vi "PH_Acq_ms.vi"(2 "PH_Settings_Params":T1={"SyncDiv"=1, "DeviceIndex"=0, "CFD0 level"=50, "CFD0 zero X"=10, "CFD1 level"=50, "CFD1 zero X"=10, "Range No."=0, "StopOnOverflow"=FALSE, "AcqTime (ms)"=0.0} {"Range No." min=0 max=5 step=1; "CFD1 zero X" min=0 max=40 step=1; "CFD1 level" min=0 max=400 step=1; "CFD0 zero X" min=-1300 max=400 step=10; "CFD0 level" min=-1300 max=400 step=10; "SyncDiv" min=1 max=8 step=1}, 3 "Deviceindex":i32, 4 "Calib Error":bool, 5 "Initialization Error":bool) -> (0 "CH1MeanRate":dbl format="%0.2f", 1 "SyncMeanRate":dbl format="%0.2f")   [LabVIEW 2019]
uses:
  <vilib>/Analysis/baseanly.llb/Mean (DBL).vi
  phlib64.dll
  <vilib>/Analysis/NI_AALBase.lvlib
panel:
  out "Elapsed Time (s)":dbl
  out "CH1Rates":i32[](array[numeric])
  out "SyncRates":i32[](array[numeric])
  out "Waveform Chart":cluster{"rate":i32}[](graph)
  out "CH1Rate":i32(slide) scale=1.0..1000000.0
  out "SyncRate":i32(slide) scale=1.0..1000000.0
  in  "stop":bool
  out "Resolution (ps)":i32
  out "PH_Settings_Error":bool
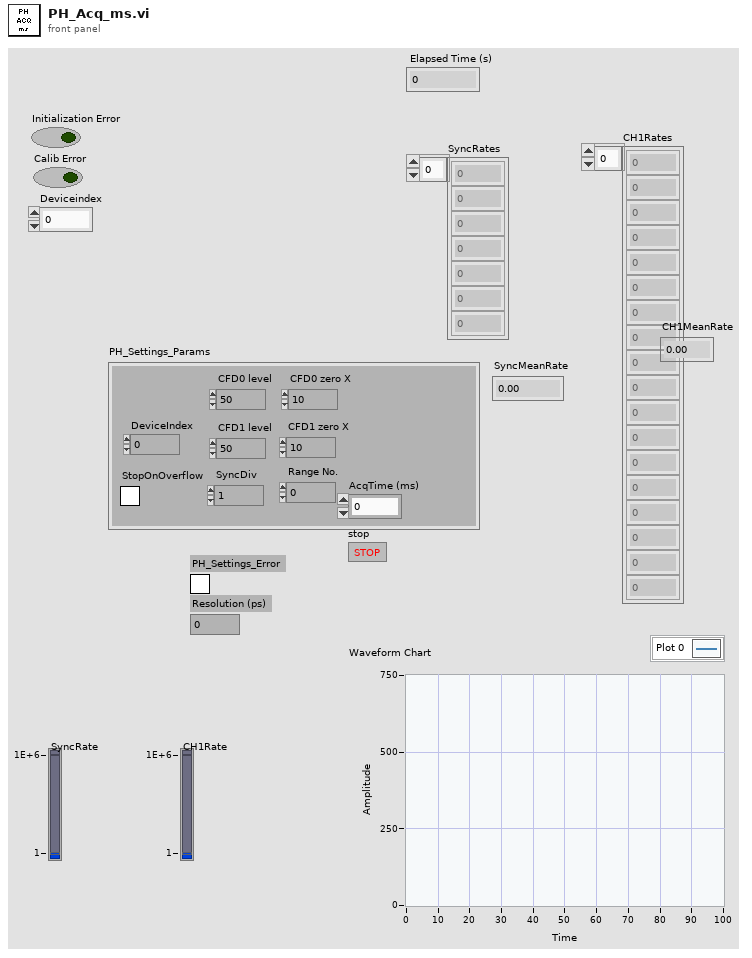
[diagram p1: front panel]
types:
  T1 = cluster{"SyncDiv":i32, "DeviceIndex":i32, "CFD0 level":i32, "CFD0 zero X":i32, "CFD1 level":i32, "CFD1 zero X":i32, "Range No.":i32, "StopOnOverflow":bool, "AcqTime (ms)":dbl}
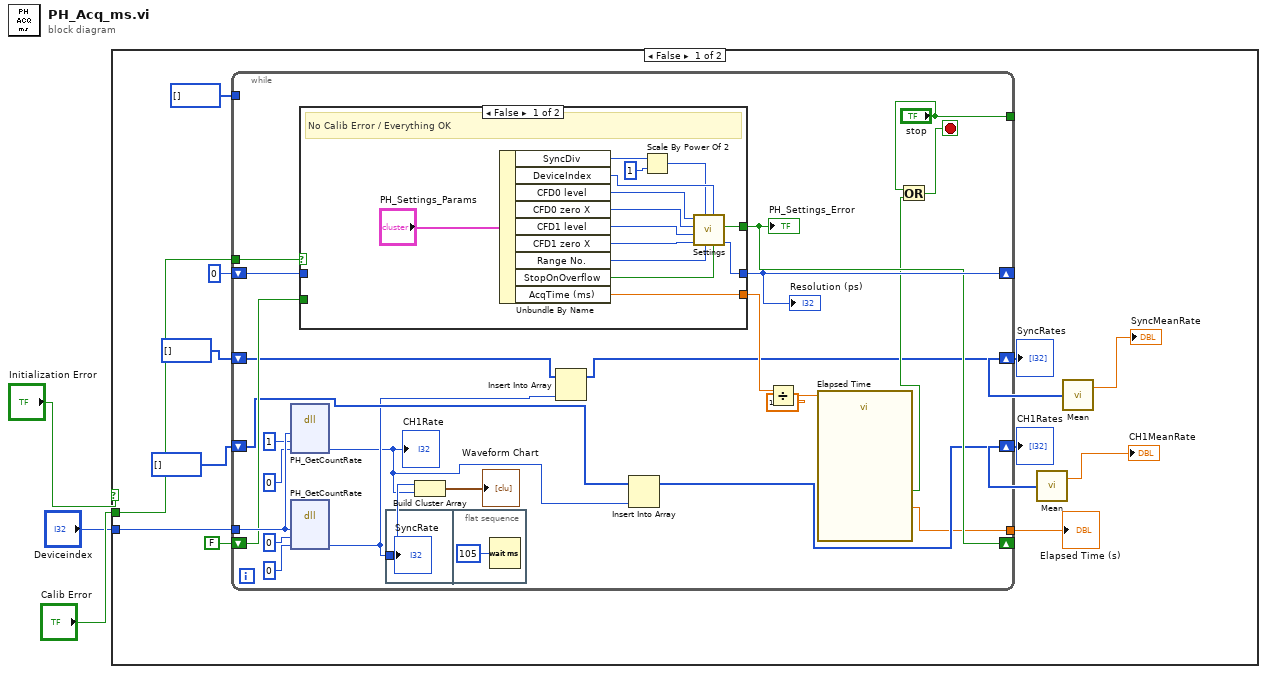
[diagram p0: block diagram]
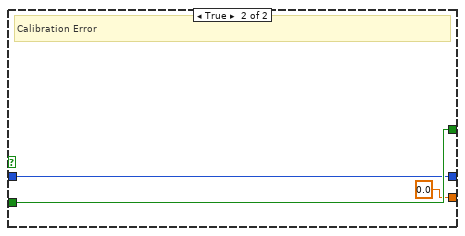
[diagram p2: hidden frame]
diagram:
  n1 = case shown="False" "Initialization Error" {
    tunnel: "Calib Error" -> [w15 _]
    tunnel: "Deviceindex" -> [w14 _]
    frame False {
      n2 = while {
        tunnel: w14 -> [w38]
        shift-right: [w33] -> _
        shift-left: 0 ("Resolution") -> [w30]
        tunnel: w15 -> [w39]
        shift-right: [w32] -> _
        shift-left: FALSE ("Error") -> [w31]
        tunnel: ["stop"] -> _
        tunnel: i32[] [] -> [_]
        shift-right: [w18] -> w8
        shift-left: i32[] [] -> [w22]
        shift-right: [w17] -> w7
        shift-left: i32[] [] -> [w21]
        tunnel: [w16] -> w4
        stop <- w25 stop-if-true
        n3 = dll-call lib="C:/Users/manip/Documents/Controle_Manip_2020/subVIs/PicoHarp/PHLib64.dll" fn="PH_GetCountRate"("devidx"=w38, "channel"=1, "rate"=0) -> ("rate"=w19:i32)  [unwired: 6 in, 2 out]
        "CH1Rate" <- w19
        n4 = dll-call lib="C:/Users/manip/Documents/Controle_Manip_2020/subVIs/PicoHarp/PHLib64.dll" fn="PH_GetCountRate"("devidx"=w38, "channel"=0, "rate"=0) -> ("rate"=w20:i32)  [unwired: 6 in, 2 out]
        n5 = case shown="False" w39 {
          tunnel: [w44 w58] -> w32
          tunnel: [w43 w57] -> w33
          tunnel: w31 -> [_ w58]
          tunnel: w30 -> [_ w57]
          tunnel: [w42 0.0 ("AcqTime (ms)")] -> w27
          frame False {
            # "No Calib Error / Everything OK"
            n6 = Unbundle By Name("PH_Settings_Params") -> ("SyncDiv"=w46:i32, "DeviceIndex"=w54:i32, "CFD0 level"=w53:i32, "CFD0 zero X"=w52:i32, "CFD1 level"=w51:i32, "CFD1 zero X"=w50:i32, "Range No."=w49:i32, "StopOnOverflow"=w48:bool, "AcqTime (ms)"=w42:dbl)
            n7 = Scale By Power Of 2(n=w46, x=1) -> (x*2^n=w47:i32)
            n8 = call "Settings.vi"("StopOnOverflow"=w48, "DeviceIndex"=w54, "Range No."=w49, "SyncDiv"=w47, "CFD1 zero X"=w50, "CFD1 level"=w51, "CFD0 zero X"=w52, "CFD0 level"=w53) -> ("Resolution"=w43:i32, "Error"=w44:bool)  [unwired: 2 in]
          }
          frame True {
            # "Calibration Error"
          }
        }
        "PH_Settings_Error" <- w32
        "Resolution (ps)" <- w33
        n9 = flat-sequence {
          tunnel: w20 -> [w40]
          frame #0 {
            "SyncRate" <- w40
          }
          frame #1 {
            n10 = Wait (ms)(milliseconds to wait=u32 105) -> ()  [unwired: 1 out]
          }
        }
        n11 = Build Cluster Array(w20, w19) -> (→"Waveform Chart":cluster{"rate":i32}[])
        n12 = Insert Into Array(array=w22, new element=w20) -> (w18:i32[])  [unwired: 1 in]
        n13 = Insert Into Array(array=w21, new element=w19) -> (w17:i32[])  [unwired: 1 in]
        n14 = Divide(x=w27, y=1000.0) -> (x/y=w26:dbl)
        n15 = call "Elapsed Time"("Time Target (s)"=w26) -> ("Elapsed Time (s)"=w16:dbl, "Time has Elapsed"=w23:bool)  [unwired: 11 in, 6 out]
        n16 = Or(x="stop", y=w23) -> (x .or. y?=w25:bool)
      }
      "SyncRates" <- w8
      "CH1Rates" <- w7
      "Elapsed Time (s)" <- w4
      n17 = call-poly <vilib>:"Mean.vi"("X"=w7) -> ("mean"=→"CH1MeanRate":dbl)  [unwired: 1 out]
      n18 = call-poly <vilib>:"Mean.vi"("X"=w8) -> ("mean"=→"SyncMeanRate":dbl)  [unwired: 1 out]
    }
    frame True {
    }
  }
